vi "rqcAlice Close KeyNET.vi"(8 "error in":errorcluster, 11 "rqcAlice ServiceNET in":T1) -> (0 "error out":errorcluster)   [LabVIEW 2016]
uses:
  Custom Controls/rqcAlice KeyNET control.ctl
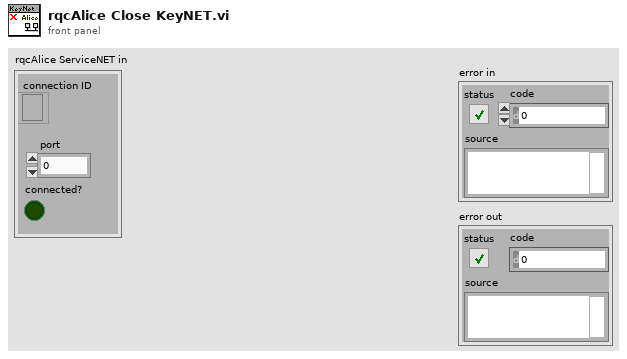
[diagram p1: front panel]
types:
  T1 = typedef "rqcAlice KeyNET control.ctl" = cluster{"connection ID":refnum<k5>, "port":u16, "connected?":bool}
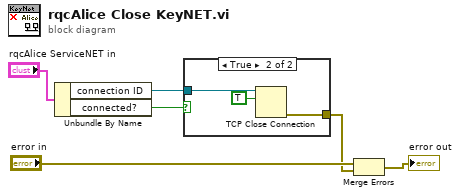
[diagram p0: block diagram]
diagram:
  n1 = Unbundle By Name("rqcAlice ServiceNET in") -> ("connection ID"=w4:refnum<k5>, "connected?"=w5:bool)
  n2 = case shown="True" w5 {
    tunnel: w4 -> [_ w9]
    tunnel: [_ w8] -> w1
    frame False {
    }
    frame True {
      n3 = TCP Close Connection(connection ID=w9, abort (F)=TRUE) -> (error out=w8:errorcluster)  [unwired: 1 in, 1 out]
    }
  }
  n4 = Merge Errors("error in", w1) -> (→"error out":errorcluster)
